vi "Read_DO.vi"() -> ()   [LabVIEW 2016]
uses:
  <vilib>/NI/Current Value Table/DataTypes/Boolean_Read.vi
  <vilib>/NI/Current Value Table/Type to Enum.vi
  <vilib>/NI/Current Value Table/DataTypes/Boolean_Type To Enum.vi
  <vilib>/Utility/file.llb/Read Delimited Spreadsheet (string).vi
  <vilib>/NI/Current Value Table/FGVs/CVT Globals.vi
  <vilib>/NI/Current Value Table/FGVs/Tag Memory.vi
  <vilib>/NI/Current Value Table/Memory Block.vi
  <vilib>/NI/Current Value Table/DataTypes/Boolean_Memory Block.vi
  <vilib>/NI/Current Value Table/Current Value Table.lvlib
panel:
  in  "stop":bool
  out "?":cluster{bool}[](array[cluster])
  out "?":cluster{bool}[](array[cluster])
  # "DOORS &\n                                 STATUS"
  # "Doctor Entrance Door-1 Open Cmd"
  # "Ist O.T.-Occupied Lamp Green"
  # "Doctor Entrance -Door-2 Open Cmd"
  # "Ist O.T-AHU Start Coil"
  # "Doctor Entrance -Hand Santizier Coil"
  # "2nd O.T.:Scrubber Dispense Coil"
  # "Main Entrance-Door Open Cmd"
  # "2nd O.T.-Door Open Cmd"
  # "OT Entrance-Door Open  Cmd"
  # "Spare D0-1"
  # "O.T Entrance-Hand Santiizier Coil"
  # "Spare D0-2"
  # "Ist O.T.- Door Open Cmd"
  # "Spare D0-3"
  # "Ist O.T-Occupied Lamp(Red)"
  # "Spare D0-4"
  # "Ist O.T-Inside Light"
  # "Spare D0-5"
  # "Ist O.T.-Scrubber Dispense Coil"
  # "Spare Do-6"
  # "DOORS &\n                    STATUS"
  # "Doctor Entrance Door-1 Open Cmd"
  # "Ist O.T.-Occupied Lamp Green"
  # "Doctor Entrance -Door-2 Open Cmd"
  # "Ist O.T-AHU Start Coil"
  # "Doctor Entrance -Hand Santizier Coil"
  # "2nd O.T.:Scrubber Dispense Coil"
  # "Main Entrance-Door Open Cmd"
  # "2nd O.T.-Door Open Cmd"
  # "OT Entrance-Door Open  Cmd"
  # "Spare DO-1"
  # "O.T Entrance-Hand Santiizier Coil"
  # "Spare DO-2"
  # "Ist O.T.- Door Open Cmd"
  # "Spare DO-3"
  # "Ist O.T-Occupied Lamp(Red)"
  # "Spare DO-4"
  # "Ist O.T-Inside Light"
  # "Spare DO-5"
  # "Ist O.T.-Scrubber Dispense Coil"
  # "Spare DO-6"
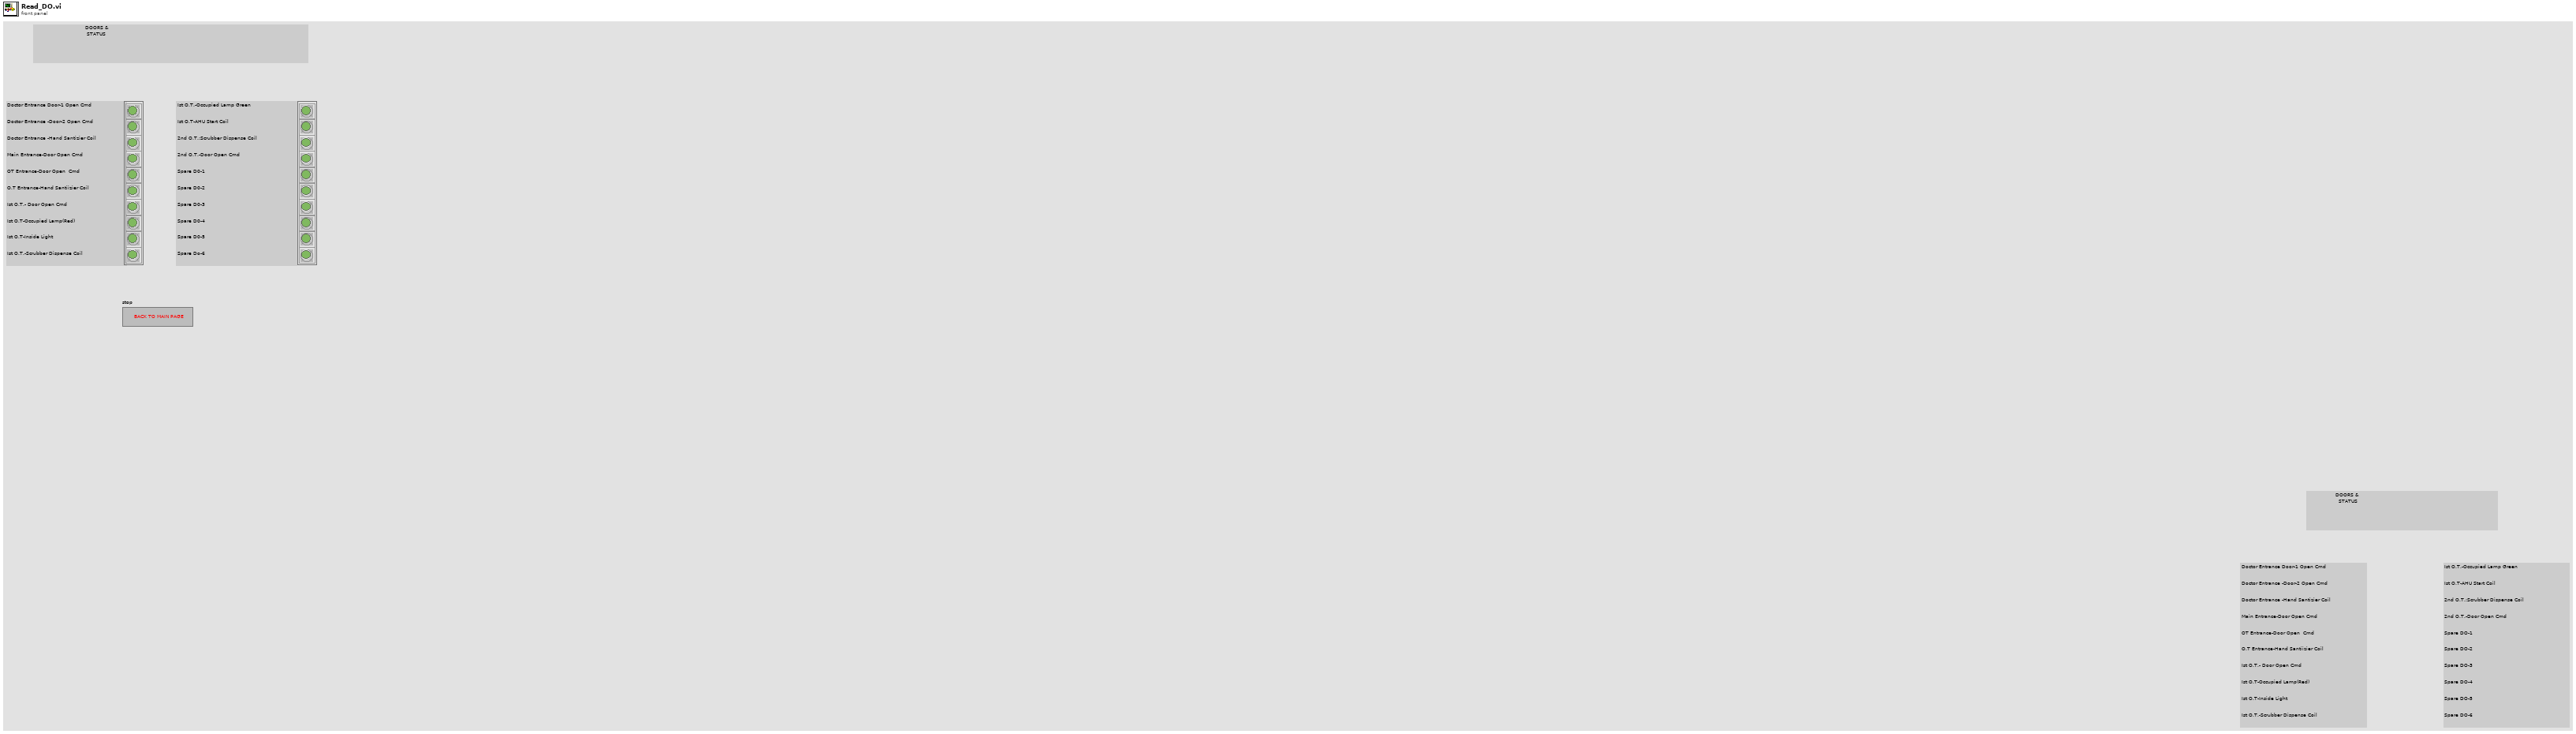
[diagram p1: front panel]
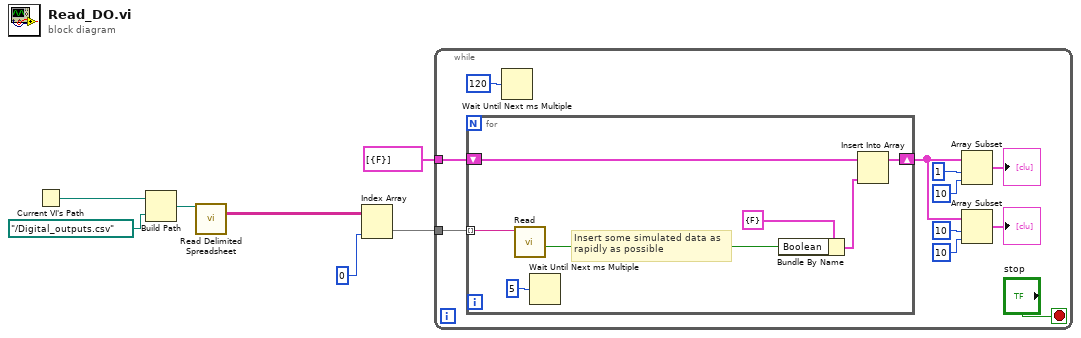
[diagram p0: block diagram]
diagram:
  n1 = Current VI's Path() -> (path=w3:path)
  n2 = Build Path(base path=w3, name or relative path=path "../Digital_outputs.csv") -> (appended path=w1:path)
  n3 = call-poly <vilib>:"Read Delimited Spreadsheet.vi"("file path (dialog if empty)"=w1) -> ("all rows"=w6:string[][])  [unwired: 9 in, 5 out]
  n4 = Index Array "Index Array"(array=w6, index (col)=0 ("disabled index (col)")) -> (element=w4:string[])  [unwired: 1 in]
  n5 = while {
    tunnel: cluster{"Boolean":bool}[] [{"Boolean"=FALSE}] ("output array") -> [w18]
    tunnel: w4 -> [w17]
    stop <- "stop" stop-if-true
    n6 = for {
      shift-right: [w22] -> w12
      shift-left: w18 -> [w23]
      tunnel: w17 -> [w21] mode=indexing
      # "Insert some simulated data as\nrapidly as possible"
      n7 = call-poly <vilib>:"Read.vi"("Tag Name"=w21) -> ("Value"=w20:bool)  [unwired: 9 in, 1 out]
      n8 = Wait Until Next ms Multiple(millisecond multiple=u32 5 ("millisecond timer value")) -> ()  [unwired: 1 out]
      n9 = Bundle By Name(cluster=cluster{"Boolean":bool} {"Boolean"=FALSE} ("Cluster"), "Boolean"=w20) -> (w24:cluster{"Boolean":bool})
      n10 = Insert Into Array(array=w23, new element=w24) -> (w22:cluster{"Boolean":bool}[])  [unwired: 1 in]
    }
    n11 = Wait Until Next ms Multiple(millisecond multiple=u32 120 ("milliseconds to wait")) -> ()  [unwired: 1 out]
    n12 = Array Subset(array=w12, index=1, length=10) -> (→"?":cluster{"Boolean":bool}[])
    n13 = Array Subset(array=w12, index=10, length=10) -> (→"?":cluster{"Boolean":bool}[])
  }
